vi "Create ResourceIn Controls and Wire Unbundler.vi"(0 "NodeIn":refnum<vi>, 5 "Unbundle_OutputTerm":refnum<vi>[](array[refnum]), 11 "error in (no error)":errorcluster) -> (15 "error out":errorcluster)   [LabVIEW 2021, in "Converter.lvlib"]
uses:
  Converter.lvlib
  Path Functions/Path Functions.lvlib
  Converter Reusables/Converter Reusables.lvlib
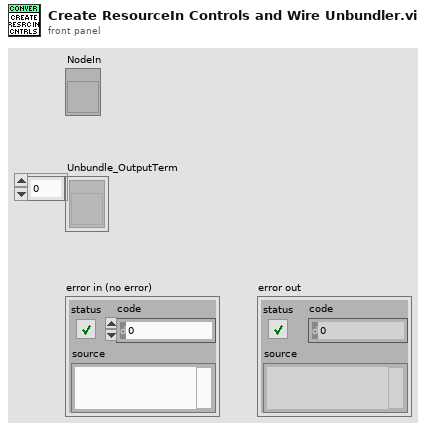
[diagram p1: front panel]
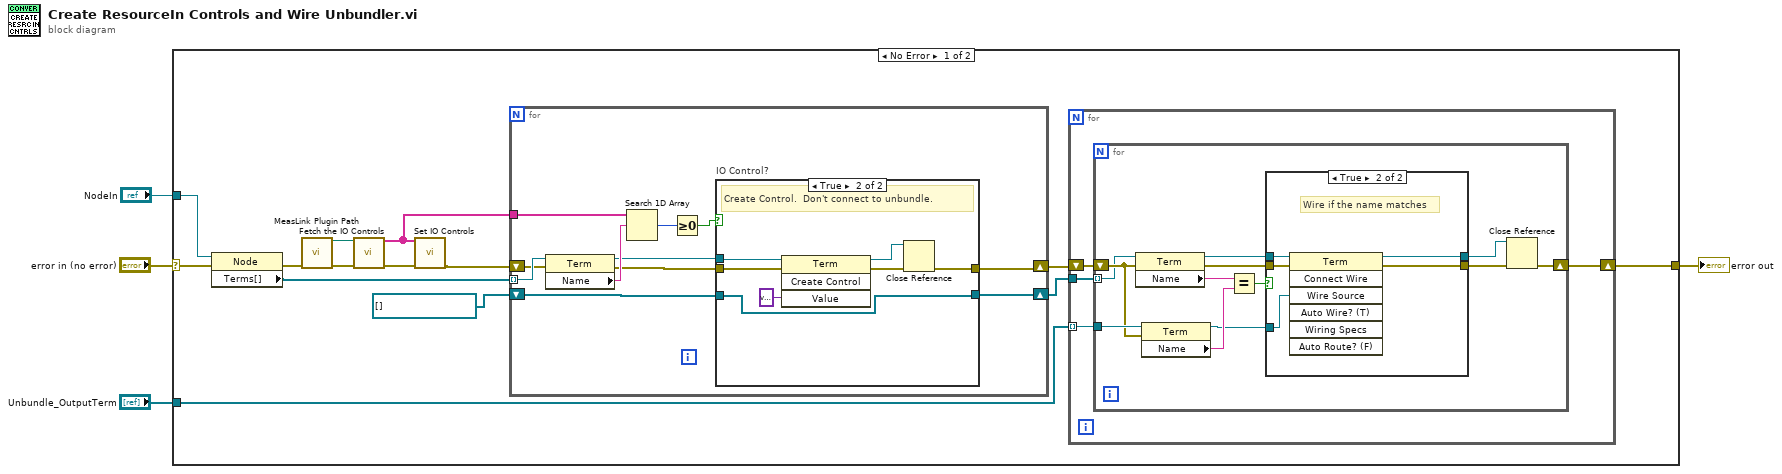
[diagram p0: block diagram]
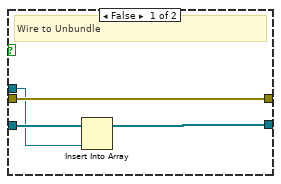
[diagram p2: hidden frame]
diagram:
  n1 = case shown="No Error" "error in (no error)" {
    selector: "error in (no error)" -> [w16 w64]
    tunnel: [w6 w64] -> w3
    tunnel: "Unbundle_OutputTerm" -> [w18 _]
    tunnel: "NodeIn" -> [w17 _]
    frame No Error {
      n2 = property class="Node"(reference=w17, error in=w16) -> (error out=w15:errorcluster, "Terms[]"=w8:refnum<vi>[])  [unwired: 1 out]
      n3 = call "MeasLink Plugin Path.vi"("error in (no error)"=w15) -> ("New Code Module"=w13:path, "error out"=w14:errorcluster)  [unwired: 2 in, 11 out]
      n4 = call "Fetch the IO Controls.vi"("VI Path"=w13, "error in (no error)"=w14) -> ("IO Controls[]"=w11:string[], "error out"=w12:errorcluster)  [unwired: 12 in]
      n5 = call "Set IO Controls.vi"("IO Controls[]"=w11, "error in (no error)"=w12) -> ("error out"=w9:errorcluster)  [unwired: 13 in]
      n6 = for {
        tunnel: w8 -> [w29] mode=indexing
        tunnel: w11 -> [w26]
        shift-right: [w21] -> w7
        shift-left: refnum<vi>[] [] -> [w20]
        shift-right: [w19] -> w10
        shift-left: w9 -> [w28]
        n7 = property class="Term"(reference=w29, error in=w28) -> (reference out=w23:refnum<vi>, error out=w22:errorcluster, "Name"=w25:string)
        n8 = Search 1D Array(1D array=w26, element=w25) -> (index of element=w27:i32)  [unwired: 1 in]
        n9 = Greater Or Equal To 0?(x=w27) -> (x >= 0?=w24:bool)
        n10 = case "IO Control?" shown="True" w24 {
          tunnel: w22 -> [w33 w40]
          tunnel: [w33 w36] -> w19
          tunnel: w23 -> [w30 w37]
          tunnel: [w31 w34] -> w21
          tunnel: w20 -> [w32 w34]
          frame False {
            # "Wire to Unbundle"
            n11 = Insert Into Array(array=w32, new element=w30) -> (w31:refnum<vi>[])  [unwired: 1 in]
          }
          frame True {
            # "Create Control.  Don't connect to unbundle."
            n12 = invoke class="Term" method="Create Control"(reference=w37, error in=w40, "Value"=variant) -> (reference out=w35:refnum<vi>, error out=w39:errorcluster)  [unwired: 1 in, 2 out]
            n13 = Close Reference(reference=w35, error in (no error)=w39) -> (error out=w36:errorcluster)
          }
        }
      }
      n14 = for {
        tunnel: w7 -> [w42]
        tunnel: w18 -> [w41] mode=indexing
        shift-right: [w43] -> w6
        shift-left: w10 -> [w44]
        n15 = for {
          tunnel: w42 -> [w53] mode=indexing
          tunnel: w41 -> [w55]
          shift-right: [w56] -> w43
          shift-left: w44 -> [w54]
          n16 = property class="Term"(reference=w53, error in=w54) -> (reference out=w51:refnum<vi>, error out=w50:errorcluster, "Name"=w46:string)
          n17 = property class="Term"(reference=w55, error in=w54) -> (reference out=w49:refnum<vi>, "Name"=w52:string)  [unwired: 1 out]
          n18 = Equal?(x=w46, y=w52) -> (x = y?=w45:bool)
          n19 = case shown="True" w45 {
            tunnel: w51 -> [w58 w63]
            tunnel: w50 -> [w57 w60]
            tunnel: w49 -> [_ w62]
            tunnel: [w57 w61] -> w48
            tunnel: [w58 w59] -> w47
            frame False {
              # "Ignore"
            }
            frame True {
              # "Wire if the name matches"
              n20 = invoke class="Term" method="Connect Wire"(reference=w63, error in=w60, "Wire Source"=w62) -> (reference out=w59:refnum<vi>, error out=w61:errorcluster)  [unwired: 4 in, 5 out]
            }
          }
          n21 = Close Reference(reference=w47, error in (no error)=w48) -> (error out=w56:errorcluster)
        }
      }
    }
    frame Error {
    }
  }
  "error out" <- w3
